vi "RSZVB Get Virtual Transform Balanced Circuit Model.vi"(7 "Logical Port Number (1)":i32=1, 8 "error in (no error)":errorcluster {"code" format="%.0x"}, 9 "Function Type (0: Deembedding)":i32(ring) items=["Deembedding", "Embedding"], 10 "Channel (1)":i32=1, 11 "VISA session":refnum<visa-resource-name>) -> (0 "error out":errorcluster {"code" format="%.0x"}, 2 "Circuit Model":i32, 3 "dup VISA session":refnum<visa-resource-name>)   [LabVIEW 2011]
doc: "This VI returns the circuit model for balanced port deembedding/embedding.\n\nRemote-control command(s):\nCALCulate<Ch>:TRANsform:VNETworks:BALanced:DEEMbedding<Log_pt>:TNDefinition?\nCALCulate<Ch>:TRANsform:VNETworks:BALanced:EMBedding<Log_pt>:TNDefinition?"
uses:
  _utility/RSZVB Global Data.vi
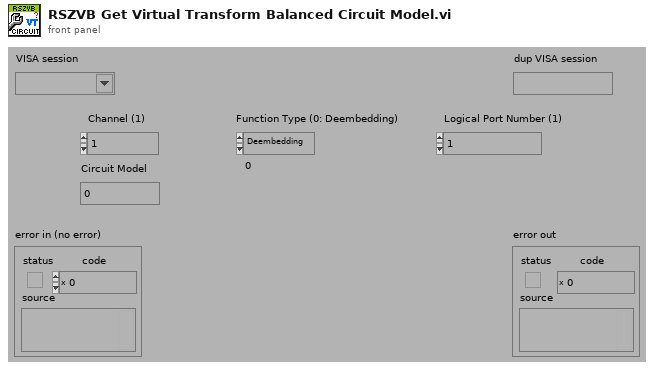
[diagram p1: front panel]
types:
  T1 = cluster{"Error Checking (T: On)":bool, "Installed Options":string[], "Data Valid?":bool, "Ports":i32, "Model":string[], "Option Checking (T: On)":bool}[]
  T2 = cluster{"Error Checking (T: On)":bool, "Installed Options":string[], "Data Valid?":bool, "Ports":i32, "Model":string[], "Option Checking (T: On)":bool}
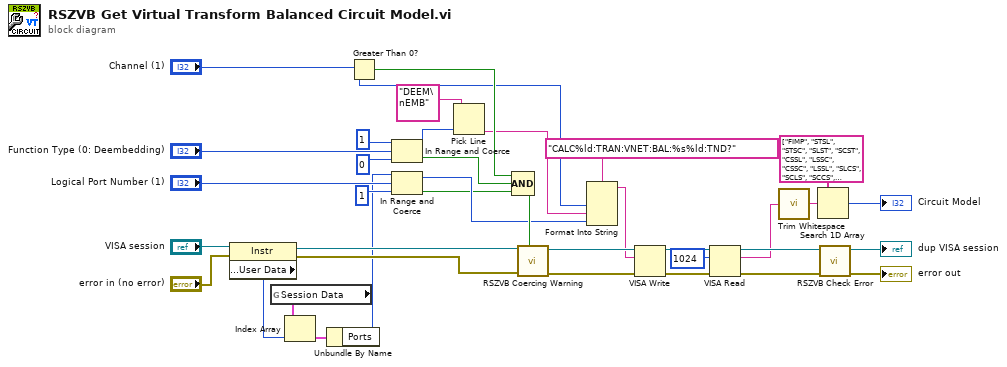
[diagram p0: block diagram]
diagram:
  n1 = property class="Instr"(reference="VISA session", error in="error in (no error)") -> (reference out=w29:refnum<visa-resource-name>, error out=w30:errorcluster, "General Settings:User Data"=w33:u32)
  n2 = global read "RSZVB Global Data.vi" "Session Data"() -> (w32:T1)
  n3 = Index Array(array=w32, index=w33) -> (element=w31:T2)
  n4 = Unbundle By Name(w31) -> ("Ports"=w12:i32)
  n5 = Greater Than 0?(x="Channel (1)") -> (x > 0?=w26:bool)
  n6 = In Range and Coerce(upper limit=1 ("lower limit"), x="Function Type (0: Deembedding)", lower limit=0) -> (coerced(x)=w20:i32, In Range?=w23:bool)
  n7 = In Range and Coerce(upper limit=w12, x="Logical Port Number (1)", lower limit=1) -> (coerced(x)=w22:i32, In Range?=w18:bool)
  n8 = Pick Line(multi-line string="DEEM\nEMB", line index=w20) -> (output string=w19:string)  [unwired: 1 in]
  n9 = Compound Arithmetic op=AND(w26, w23, w18) -> (w25:bool)
  n10 = call "RSZVB Coercing Warning.vi"("In Range?"=w25, "error in (no error)"=w30, "VISA session"=w29) -> ("error out"=w36:errorcluster, "dup VISA session"=w37:refnum<visa-resource-name>)  [unwired: 7 in]
  n11 = Format Into String(format string="CALC%ld:TRAN:VNET:BAL:%s%ld:TND?", "Channel (1)", w19, w22) -> (resulting string=w34:string)  [unwired: 2 in, 1 out]
  n12 = VISA Write(VISA resource name=w37, write buffer=w34, error in (no error)=w36) -> (VISA resource name out=w4:refnum<visa-resource-name>, error out=w5:errorcluster)  [unwired: 1 out]
  n13 = VISA Read(VISA resource name=w4, byte count=u32 1024 ("byte count (0)"), error in (no error)=w5) -> (VISA resource name out=w10:refnum<visa-resource-name>, read buffer=w6:string, error out=w9:errorcluster)  [unwired: 1 out]
  n14 = call <vilib>:"Trim Whitespace.vi"("string"=w6) -> ("trimmed string"=w7:string)  [unwired: 1 in]
  n15 = Search 1D Array(1D array=string[] ["FIMP", "STSL", "STSC", "SLST", "SCST", "CSSL", "LSSC", "CSSC", "LSSL", "SLCS", "SCLS", "SCCS", "SLLS"] ("array 2"), element=w7) -> (index of element=→"Circuit Model":i32)  [unwired: 1 in]
  n16 = call "RSZVB Check Error.vi"("error in (no error)"=w9, "VISA session"=w10) -> ("error out"=→"error out":errorcluster, "dup VISA session"=→"dup VISA session":refnum<visa-resource-name>)  [unwired: 8 in]
